vi "Input Check.vi"   [LabVIEW 2020]
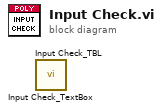
[diagram p0: block diagram]
diagram:
  n1 = call "Input Check_TextBox.vi"() -> ()  [unwired: 9 in, 3 out]
  n2 = call "Input Check_TBL.vi"() -> ()  [unwired: 8 in, 4 out]
